vi "Load Devices.vi"(8 "error in (no error)":errorcluster, 9 "device":refnum<class "Device.lvclass">[](array[class]), 10 "Device Manager in":refnum<class "Device Manager.lvclass">, 11 "Caller Actor in":refnum<class "Actor.lvclass">) -> (0 "error out":errorcluster, 3 "Caller Actor out":refnum<class "Actor.lvclass">)   [LabVIEW 2023, in "Device Manager.lvclass"]
uses:
  Device Manager.lvclass
  Device/Device/Device.lvclass
  C:/Program Files (x86)/National Instruments/LabVIEW 2023/vi.lib/ActorFramework/Actor/Actor.lvclass
  <vilib>/ActorFramework/Actor/Actor.lvclass
  Device Manager.lvclass/Device Manager.ctl
  Device/Device/Device.lvclass/Device.ctl
  <vilib>/ActorFramework/Message Enqueuer/Message Enqueuer.lvclass/Message Enqueuer.ctl
  Device/Device/Accessor/Get Device Name.vi
  <vilib>/ActorFramework/Message Enqueuer/Enqueue.vi
  Device/Device Messages/Load Action Msg/Load Action Msg.lvclass
  C:/Program Files (x86)/National Instruments/LabVIEW 2023/vi.lib/ActorFramework/Message/Message.lvclass
  Device/Device Messages/Configure Action Msg/Configure Action Msg.lvclass
  Device/Device Messages/Start Action Msg/Start Action Msg.lvclass
  <vilib>/ActorFramework/Message Priority Queue/Priority Enqueue.vi
panel:
  out "Device Manager out":refnum<class "Device Manager.lvclass">
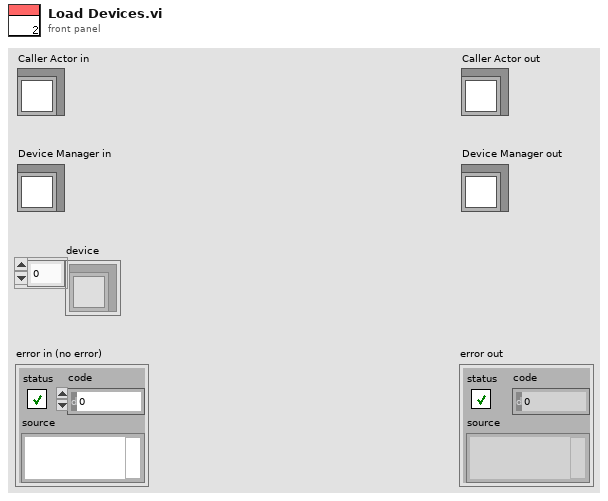
[diagram p1: front panel]
types:
  T1 = map{string, refnum<class "Message Enqueuer.lvclass">}
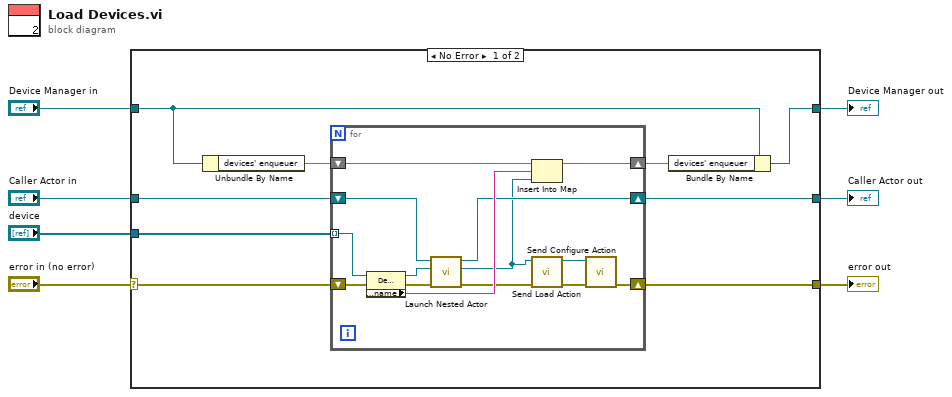
[diagram p0: block diagram]
diagram:
  n1 = case shown="No Error" "error in (no error)" {
    selector: "error in (no error)" -> [w14 w33]
    tunnel: [w9 w33] -> w6
    tunnel: [w12 w32] -> w4
    tunnel: "Device Manager in" -> [w13 w32]
    tunnel: "device" -> [w10 _]
    tunnel: "Caller Actor in" -> [w11 w31]
    tunnel: [w8 w31] -> w1
    frame No Error {
      n2 = Unbundle By Name(w13) -> ("devices' enqueuer"=w16:T1)
      n3 = for {
        tunnel: w10 -> [w23] mode=indexing
        shift-right: [w27] -> w15
        shift-left: w16 -> [w29]
        shift-right: [w17] -> w9
        shift-left: w14 -> [w25]
        shift-right: [w22] -> w8
        shift-left: w11 -> [w24]
        n4 = property class="Device.lvclass"(reference=w23, error in=w25) -> (reference out=w26:refnum<class "Device.lvclass">, error out=w30:errorcluster, "Accessor:name"=w28:string)
        n5 = call <vilib>:"Launch Nested Actor.vi"("error in (no error)"=w30, "Nested Actor"=w26, "Caller Actor in"=w24) -> ("error out"=w19:errorcluster, "Nested Actor's Enqueuer"=w18:refnum<class "Message Enqueuer.lvclass">, "Caller Actor out"=w22:refnum<class "Actor.lvclass">)  [unwired: 6 in]
        n6 = Insert Into Map(map in=w29, key=w28, value=w18) -> (map out=w27:T1)  [unwired: 2 out]
        n7 = call "Send Load Action.vi"("error in (no error)"=w19, "Message Enqueuer"=w18) -> ("error out"=w21:errorcluster, "Message Enqueuer out"=w20:refnum<class "Message Enqueuer.lvclass">)  [unwired: 8 in]
        n8 = call "Send Configure Action.vi"("error in (no error)"=w21, "Message Enqueuer"=w20) -> ("error out"=w17:errorcluster)  [unwired: 8 in, 1 out]
      }
      n9 = Bundle By Name(cluster=w13, "devices' enqueuer"=w15) -> (w12:refnum<class "Device Manager.lvclass">)
    }
    frame Error {
    }
  }
  "error out" <- w6
  "Device Manager out" <- w4
  "Caller Actor out" <- w1
